vi "Stop Core.vi"(10 "final error code":i32, 11 "Nested in":refnum<class "Interactor.lvclass">) -> (3 "Nested out":refnum<class "Interactor.lvclass">)   [LabVIEW 2024, in "Interactor.lvlib" / "Interactor.lvclass"]
doc: "(<B>Filename</B>: Actor Framework.lvlib:Actor.lvclass:Stop Core.vi)\n\nDefines what the actor does before it stops. Use the <B>final error code</B> input to determine whether the actor shut down in response to an error.\n\nBy default, this method does nothing. A descendant class may override it to define behavior, such as shutting down any processes the actor initiated in its override of the Actor Core method."
uses:
  Interactor.lvclass
  Interactor.lvclass/Interactor.ctl
  <vilib>/MGI/Panel Manager/Panel Actor/Panel Actor/Panel Actor.lvclass
  CANopen Master/CANopen Master.lvclass
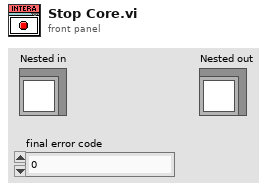
[diagram p1: front panel]
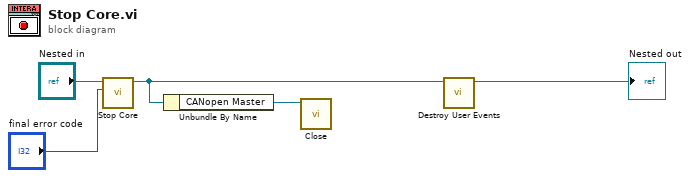
[diagram p0: block diagram]
diagram:
  n1 = call-parent "Stop Core.vi"("final error code"="final error code", "Actor in"="Nested in") -> ("Actor out"=w1:refnum<class "Interactor.lvclass">)  [unwired: 9 in]
  n2 = Unbundle By Name(w1) -> ("CANopen Master"=w2:refnum<class "CANopen Master.lvclass">)
  n3 = call "Close.vi"("CANopen Master in"=w2) -> ()  [unwired: 9 in, 2 out]
  n4 = call "Destroy User Events.vi"("UI Template in"=w1) -> ("UI Template out"=→"Nested out":refnum<class "Interactor.lvclass">)  [unwired: 10 in]
